vi "Configure Reference Channel.vi"   [LabVIEW 2018, in "Agilent MXA Series.lvlib"]
doc: "Configures the Reference Channel under Spectrum Emission Mask measurement."
uses:
  Agilent MXA Series.lvlib
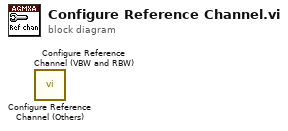
[diagram p0: block diagram]
diagram:
  n1 = call "Configure Reference Channel (Others).vi"() -> ()  [unwired: 14 in, 2 out]
  n2 = call "Configure Reference Channel (VBW and RBW).vi"() -> ()  [unwired: 14 in, 2 out]
